vi "Test_GetControlPlans.vi"() -> ()   [LabVIEW 2019]
uses:
  ByteGSAPIBase.lvclass
  ControlPlans/ControlPlan.ctl
panel:
  out "Control Plan":i32(listbox)
  out "error out":errorcluster
  out "ByteGSAPIBase out":refnum<class "ByteGSAPIBase.lvclass">
  out "Values":T1[](array[typedef])
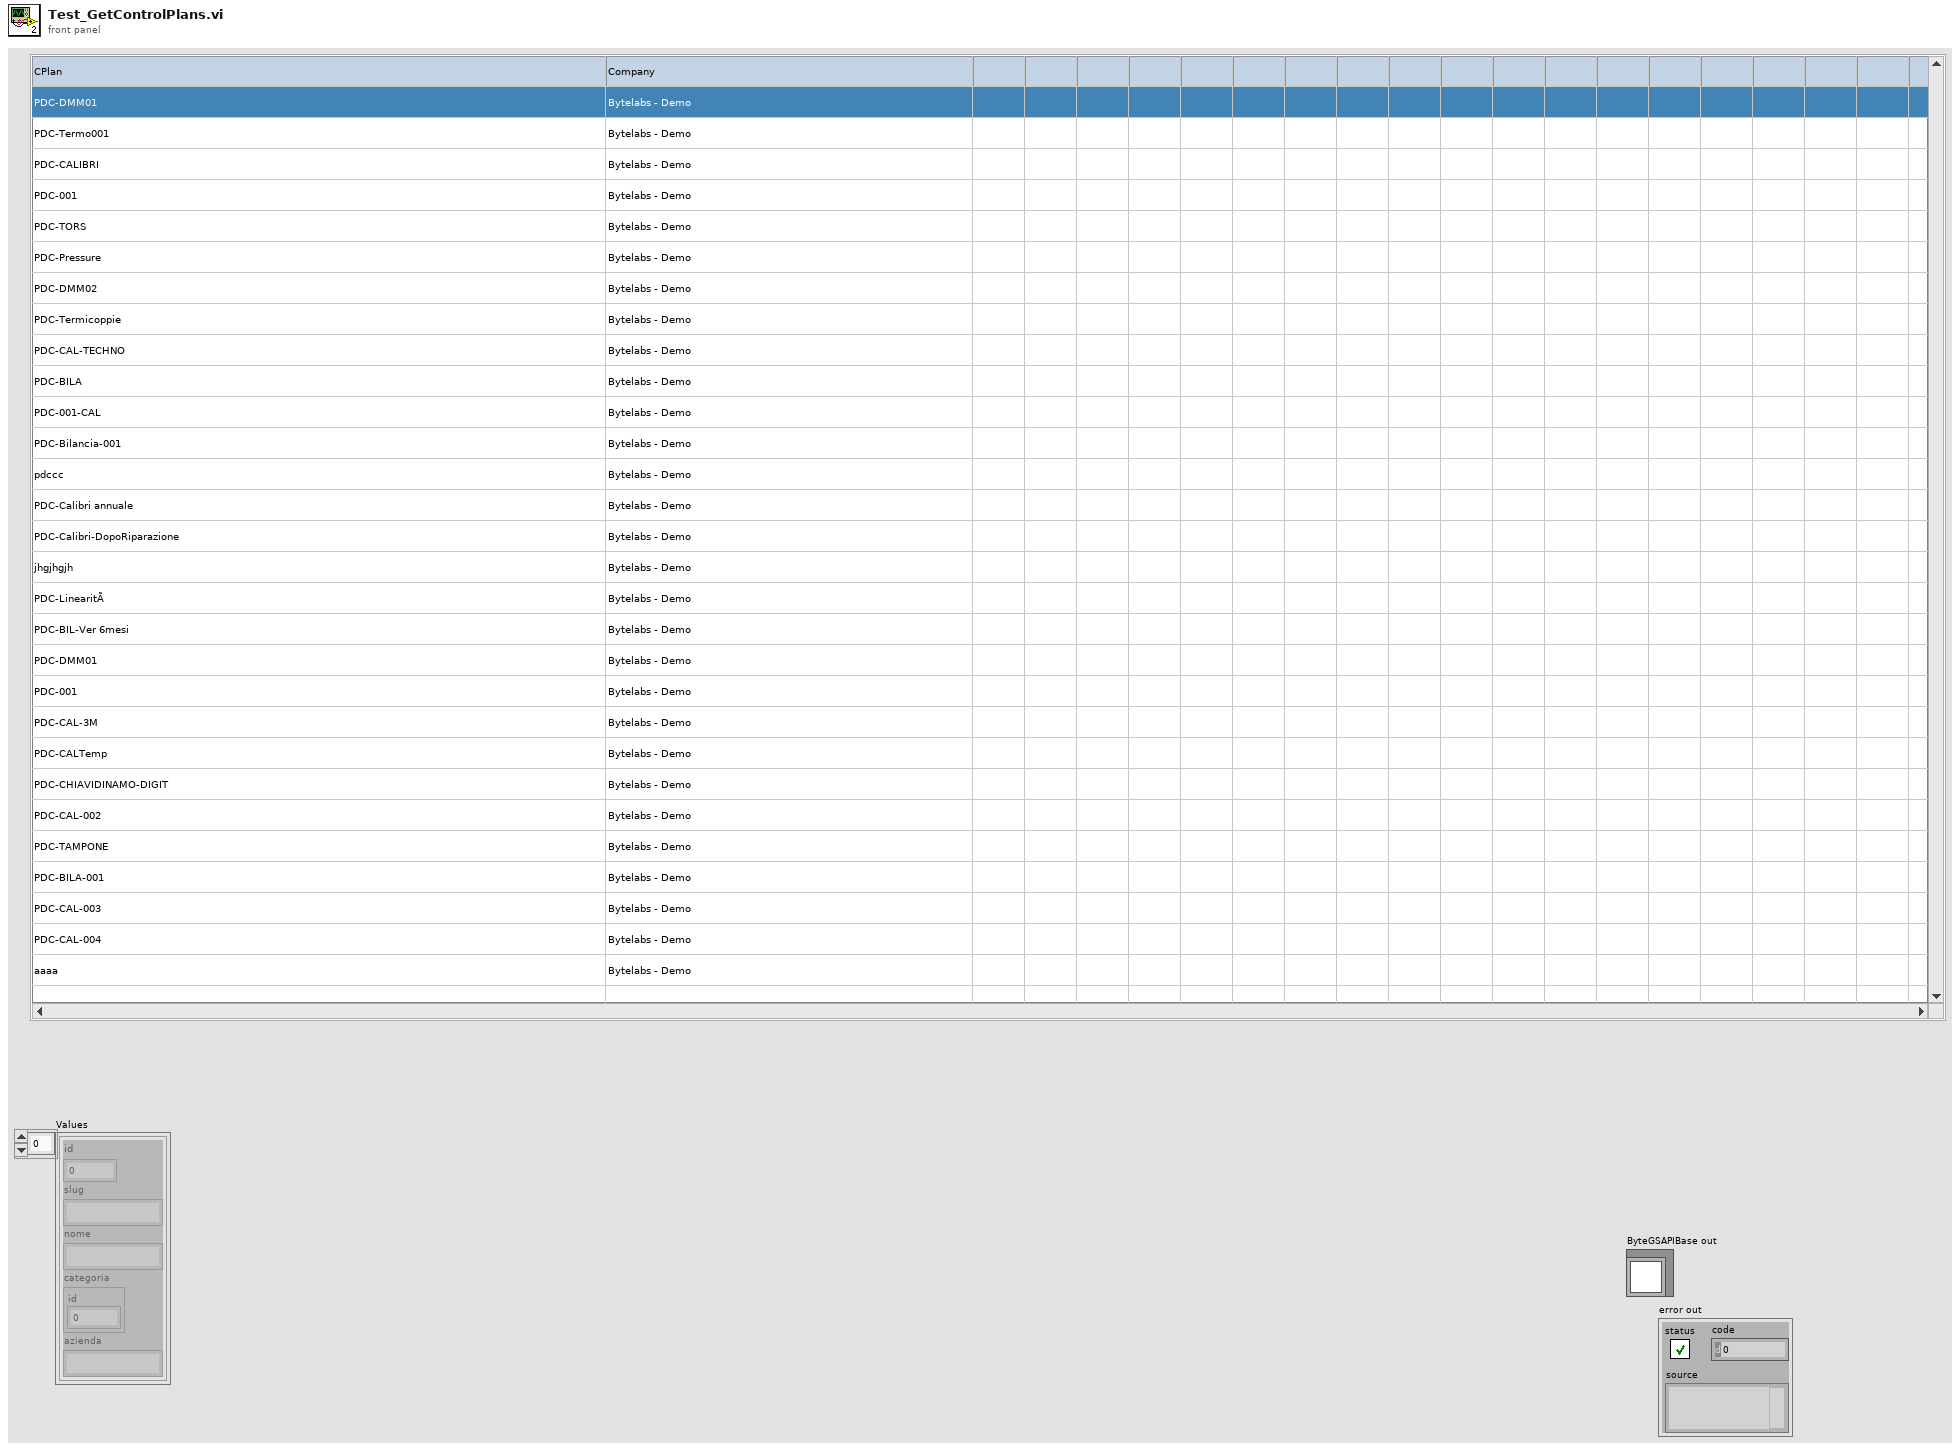
[diagram p1: front panel]
types:
  T1 = typedef "ByteGSWebAPI.lvlib/ByteGSAPIBase.lvclass/ControlPlan.ctl" = cluster{"id":i32, "slug":string, "nome":string, "categoria":cluster{"id":i32}, "azienda":string}
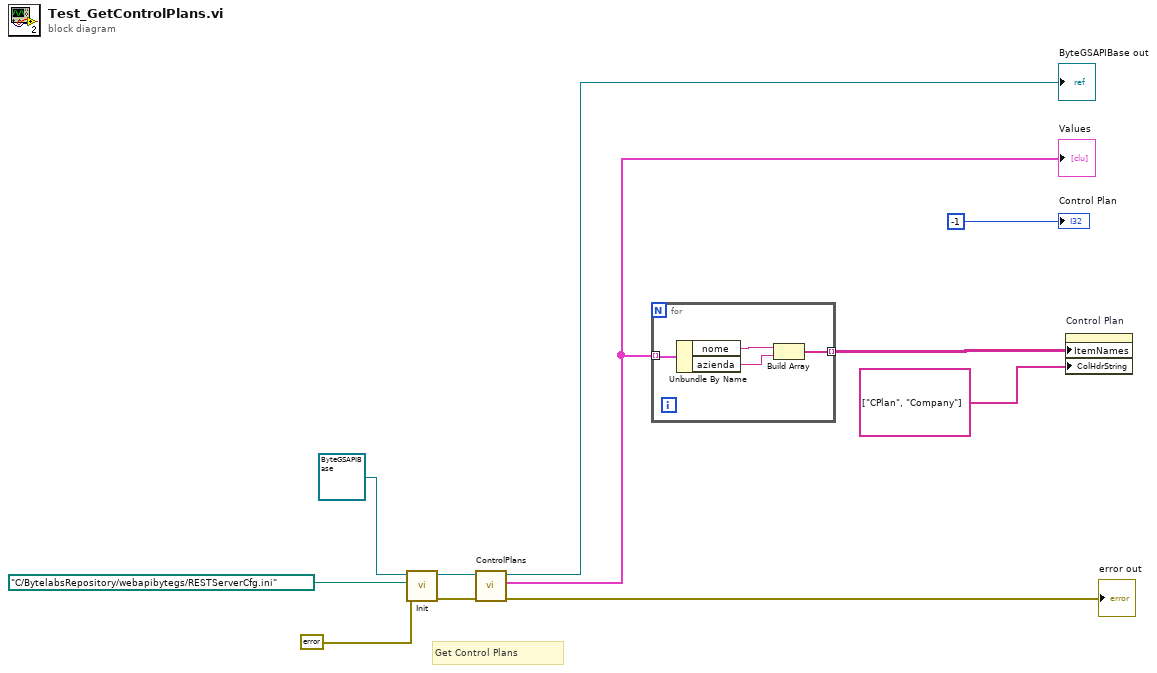
[diagram p0: block diagram]
diagram:
  # "Get Control Plans"
  n1 = call-dynamic "Init.vi"("error in (no error)"=errorcluster {"status"=FALSE, "code"=0, "source"=""}, "Server cfg"=path "C:/BytelabsRepository/webapibytegs/RESTServerCfg.ini" ("configuration file path"), "ByteGSAPIBase in"=refnum<class "ByteGSAPIBase.lvclass"> refnum) -> ("error out"=w9:errorcluster, "ByteGSAPIBase out"=w8:refnum<class "ByteGSAPIBase.lvclass">)  [unwired: 7 in]
  n2 = call-dynamic "ControlPlans.vi"("error in (no error)"=w9, "ByteGSAPIBase in"=w8) -> ("error out"=→"error out":errorcluster, "Values"=w5:T1[], "ByteGSAPIBase out"=→"ByteGSAPIBase out":refnum<class "ByteGSAPIBase.lvclass">)  [unwired: 7 in]
  "Values" <- w5
  n3 = for {
    tunnel: w5 -> [w15] mode=indexing
    tunnel: [w12] -> w4 mode=indexing
    n4 = Unbundle By Name(w15) -> ("nome"=w14:string, "azienda"=w13:string)
    n5 = Build Array(w14, w13) -> (w12:string[])
  }
  n6 = property on="Control Plan" class="MCListbox (strict)"("ItemNames"=w4, "ColHdrString"=string[] ["CPlan", "Company"] ("Column Header Strings[]")) -> ()  [unwired: 2 in, 2 out]
  "Control Plan" <- -1 ("Control Plan")
